vi "Apply Icon into VIs.vi"(7 "Substitute Layer":refnum<class "Layer.lvclass">, 8 "error in":errorcluster, 11 "VI in":refnum<vi>) -> (0 "error out":errorcluster, 3 "VI Refnum out":refnum<vi>)   [LabVIEW 2023, in "Plugin Generator.lvlib"]
uses:
  Plugin Generator.lvlib
  <vilib>/LabVIEW Icon API/lv_icon/Classes/Layer/Layer.lvclass
  <vilib>/LabVIEW Icon API/LabVIEW Icon API.lvlib
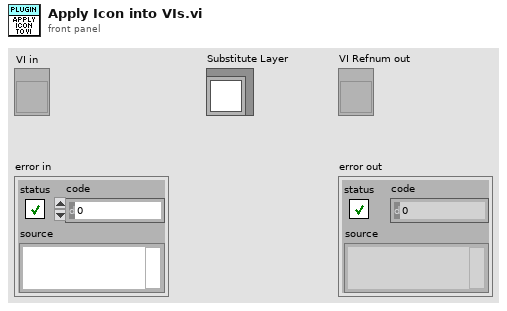
[diagram p1: front panel]
types:
  T1 = typedef "imagedata.ctl" = cluster{"image type":i32, "image depth":i32, "image":u8[], "mask":u8[], "colors":u32[], "Rectangle":cluster{"left":i16, "top":i16, "right":i16, "bottom":i16}}
  T2 = typedef "LabVIEW Icon Stored Information.ctl" = cluster{"Text Visible?":bool, "Text Opacity":u8, "Templ Visible?":bool, "Templ Opacity":u8, "Relative Path from 1 to 2":path, "Image":picture, "All User Layers":refnum<class "Layer.lvclass">[], "Body Text":T3}
  T3 = typedef "BodyText.ctl" = cluster{"Line 1 text":string, "Line 2 text":string, "Line 3 text":string, "Line 4 text":string, "Line 1 color":u32, "Line 2 color":u32, "Line 3 color":u32, "Line 4 color":u32, "Body Text Spec":cluster{"Font":T4, "Alignment":T5, "Size":u8}, "Center text vertically":bool, "Capitalize Text":bool}
  T4 = typedef "Font.ctl" = string
  T5 = typedef "Alignment.ctl" = u16
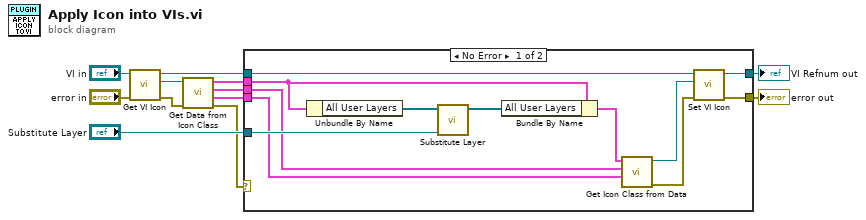
[diagram p0: block diagram]
diagram:
  n1 = call <vilib>:"Get VI Icon.vi"("error in (no error)"="error in", "VI Refnum in"="VI in") -> ("error out"=w4:errorcluster, "Icon"=w12:refnum<class "Icon.lvclass">, "VI Refnum out"=w8:refnum<vi>)  [unwired: 7 in]
  n2 = call <vilib>:"Get Data from Icon Class.vi"("error in (no error)"=w4, "Icon in"=w12) -> ("error out"=w3:errorcluster, "BW Image Data"=w6:T1, "Color Image Data"=w7:T1, "Icon data"=w9:T2)  [unwired: 6 in]
  n3 = case shown="No Error" w3 {
    selector: w3 -> [_ w25]
    tunnel: "Substitute Layer" -> [w23 _]
    tunnel: w9 -> [w22 _]
    tunnel: w8 -> [w20 w26]
    tunnel: w7 -> [w18 _]
    tunnel: w6 -> [w17 _]
    tunnel: [w15 w26] -> w5
    tunnel: [w13 w25] -> w1
    frame No Error {
      n4 = Unbundle By Name(w22) -> ("All User Layers"=w24:refnum<class "Layer.lvclass">[])
      n5 = call <vilib>:"Substitute Layer.vi"("Substitute Layer"=w23, "All User Layers in"=w24) -> ("All User Layers out"=w21:refnum<class "Layer.lvclass">[])  [unwired: 9 in]
      n6 = Bundle By Name(cluster=w22, "All User Layers"=w21) -> (w19:T2)
      n7 = call <vilib>:"Get Icon Class from Data.vi"("BW Icon"=w17, "Color Icon"=w18, "Icon Data"=w19) -> ("error out"=w14:errorcluster, "Icon out"=w16:refnum<class "Icon.lvclass">)  [unwired: 7 in]
      n8 = call <vilib>:"Set VI Icon.vi"("error in (no error)"=w14, "Icon"=w16, "VI Refnum in"=w20) -> ("error out"=w13:errorcluster, "VI Refnum out"=w15:refnum<vi>)  [unwired: 7 in]
    }
    frame Error {
    }
  }
  "VI Refnum out" <- w5
  "error out" <- w1
